vi "Insert Into Buffer.vi"(9 "Block":u8[](array[numeric]) format="%02x", 10 "Seqno":u8, 11 "Block Upload Sub-Block Transfer in":refnum<class "Block Upload Sub-Block Transfer.lvclass">) -> (3 "Block Upload Sub-Block Transfer out":refnum<class "Block Upload Sub-Block Transfer.lvclass">)   [LabVIEW 2020, in "CANopen.lvlib" / "SDO Manager.lvlib" / "Block Upload Sub-Block Transfer.lvclass"]
uses:
  Block Upload Sub-Block Transfer.lvclass
  Block Upload Sub-Block Transfer.lvclass/Block Upload Sub-Block Transfer.ctl
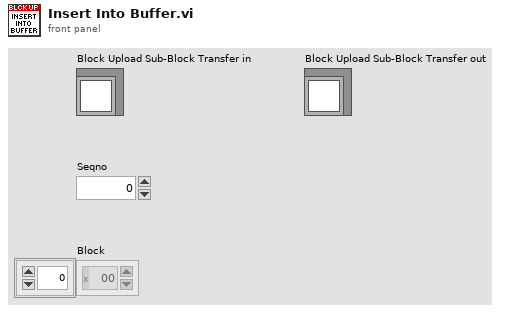
[diagram p1: front panel]
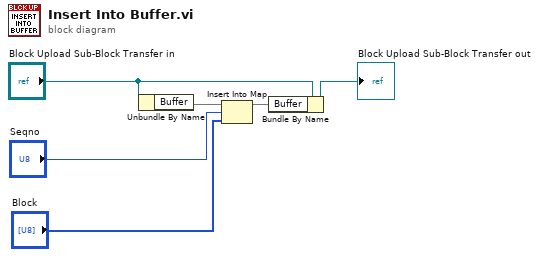
[diagram p0: block diagram]
diagram:
  n1 = Unbundle By Name("Block Upload Sub-Block Transfer in") -> ("Buffer"=w5:map{u8, u8[]})
  n2 = Insert Into Map(map in=w5, key="Seqno", value="Block") -> (map out=w1:map{u8, u8[]})  [unwired: 2 out]
  n3 = Bundle By Name(cluster="Block Upload Sub-Block Transfer in", "Buffer"=w1) -> (→"Block Upload Sub-Block Transfer out":refnum<class "Block Upload Sub-Block Transfer.lvclass">)
